vi "TA for 3.0.vi"(0 "Folder Name":string, 1 "Name of File":string, 2 "Folder to Save":path, 3 "Timepoints":dbl[](array[numeric]), 4 "Vx array":dbl, 5 "Vy array":dbl) -> ()   [LabVIEW 2015]
uses:
  <vilib>/Utility/file.llb/Read Delimited Spreadsheet (DBL).vi
  <vilib>/Utility/file.llb/Write Delimited Spreadsheet (DBL).vi
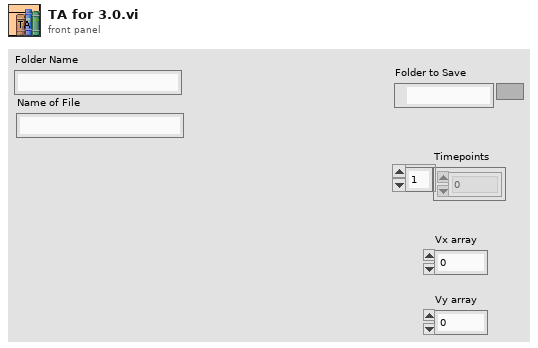
[diagram p1: front panel]
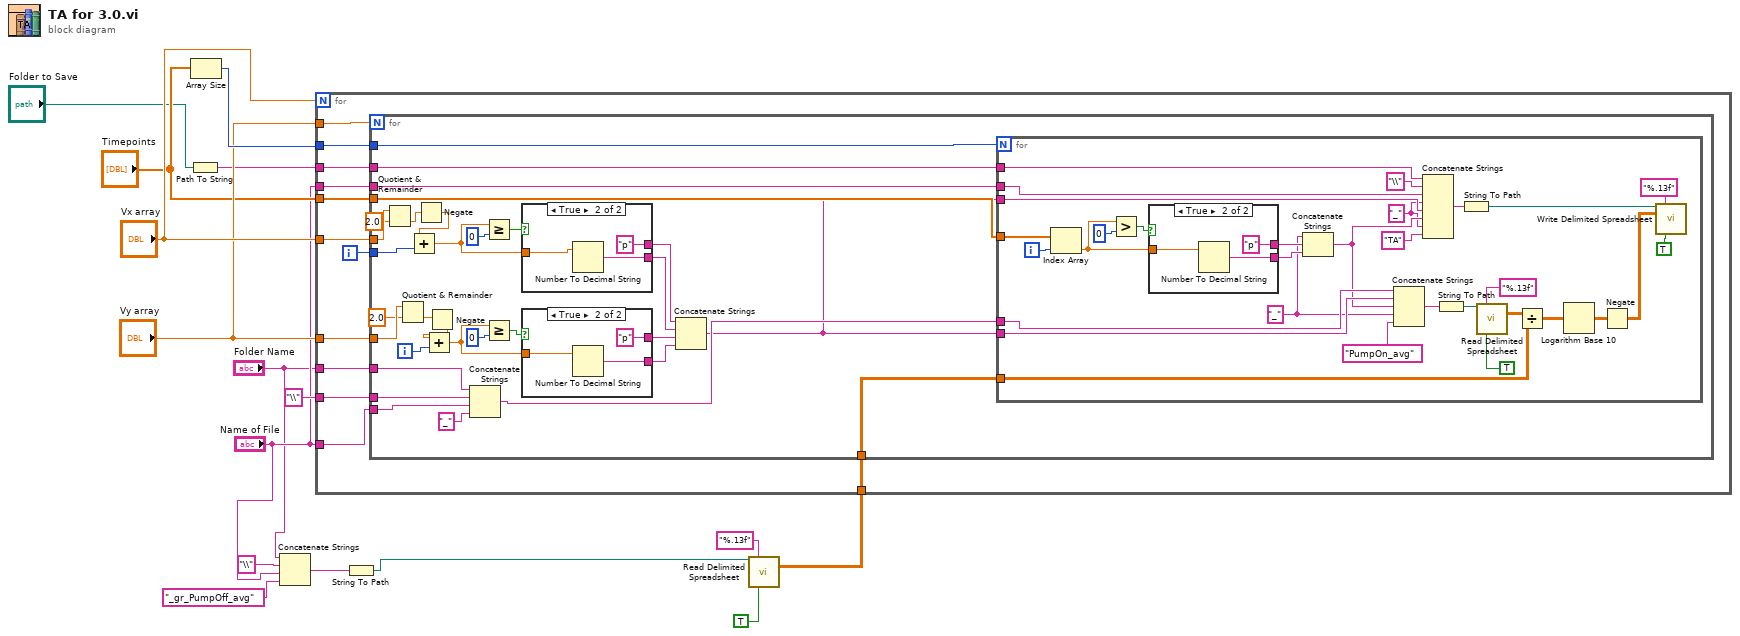
[diagram p0: block diagram]
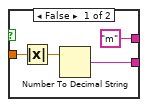
[diagram p2: hidden frame]
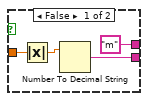
[diagram p3: hidden frame]
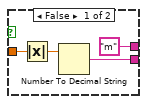
[diagram p4: hidden frame]
diagram:
  n1 = Path To String(path="Folder to Save") -> (string=w11:string)
  n2 = Array Size(array="Timepoints") -> (size(s)=w15:i32)
  n3 = Concatenate Strings("Folder Name", "\\" ("string"), "Name of File", "_gr_PumpOff_avg" ("string")) -> (w3:string)
  n4 = String To Path(string=w3) -> (path=w2:path)
  n5 = call-poly <vilib>:"Read Delimited Spreadsheet.vi"("file path (dialog if empty)"=w2, "format (%.3f)"="%.13f", "transpose? (F)"=TRUE) -> ("all rows"=w8:dbl[][])  [unwired: 7 in, 5 out]
  n6 = for {
    N: "Vx array" -> [_]
    tunnel: "Name of File" -> [w28]
    tunnel: "\\" -> [w27]
    tunnel: "Folder Name" -> [w26]
    tunnel: "Vy array" -> [w25]
    tunnel: w15 -> [w24]
    tunnel: "Vx array" -> [w23]
    tunnel: "Vy array" -> [w21]
    tunnel: "Timepoints" -> [w20]
    tunnel: w11 -> [w19]
    tunnel: "Name of File" -> [w18]
    tunnel: w8 -> [w17]
    i -> [w22]
    n7 = for {
      N: w25 -> [_]
      tunnel: w28 -> [w38]
      tunnel: w27 -> [w39]
      tunnel: w26 -> [w59]
      tunnel: w24 -> [w58]
      tunnel: w23 -> [w36]
      tunnel: w22 -> [w55]
      tunnel: w21 -> [w32]
      tunnel: w20 -> [w45]
      tunnel: w19 -> [w44]
      tunnel: w18 -> [w43]
      tunnel: w17 -> [w37]
      i -> [w50]
      n8 = Quotient & Remainder(x=w36, y=2.0) -> (floor(x/y)=w34:dbl)  [unwired: 1 out]
      n9 = Quotient & Remainder(x=w32, y=2.0) -> (floor(x/y)=w30:dbl)  [unwired: 1 out]
      n10 = Negate(x=w34) -> (-x=w33:dbl)
      n11 = Add(x=w33, y=w55) -> (x+y=w54:dbl)
      n12 = Negate(x=w30) -> (-x=w29:dbl)
      n13 = Add(x=w29, y=w50) -> (x+y=w51:dbl)
      n14 = Concatenate Strings(w59, w39, w38, "_") -> (w41:string)
      n15 = Greater Or Equal?(x=w54, y=0) -> (x >= y?=w56:bool)
      n16 = Greater Or Equal?(x=w51, y=0) -> (x >= y?=w53:bool)
      n17 = case shown="True" w56 {
        tunnel: ["m" "p"] -> w49
        tunnel: w54 -> [w69 w71]
        tunnel: [w67 w72] -> w48
        frame False {
          n18 = Absolute Value(x=w69) -> (abs(x)=w68:dbl)
          n19 = Number To Decimal String(number=w68) -> (decimal integer string=w67:string)  [unwired: 1 in]
        }
        frame True {
          n20 = Number To Decimal String(number=w71) -> (decimal integer string=w72:string)  [unwired: 1 in]
        }
      }
      n21 = case shown="True" w53 {
        tunnel: ["m" "p"] -> w47
        tunnel: w51 -> [w62 w64]
        tunnel: [w60 w65] -> w46
        frame False {
          n22 = Absolute Value(x=w62) -> (abs(x)=w61:dbl)
          n23 = Number To Decimal String(number=w61) -> (decimal integer string=w60:string)  [unwired: 1 in]
        }
        frame True {
          n24 = Number To Decimal String(number=w64) -> (decimal integer string=w65:string)  [unwired: 1 in]
        }
      }
      n25 = Concatenate Strings(w49, w48, w47, w46) -> (w40:string)
      n26 = for {
        N: w58 -> [_]
        tunnel: w45 -> [w101]
        tunnel: w44 -> [w96]
        tunnel: w43 -> [w93]
        tunnel: w41 -> [w87]
        tunnel: w40 -> [w86]
        tunnel: w37 -> [w77]
        tunnel: w40 -> [w83]
        i -> [w100]
        w85 = "_"
        w81 = "_" ("string")
        n27 = Index Array(array=w101, index=w100) -> (element=w103:dbl)
        n28 = Greater?(x=w103, y=0) -> (0:w102:bool)
        n29 = case shown="True" w102 {
          tunnel: ["m" "p"] -> w98
          tunnel: w103 -> [w107 w109]
          tunnel: [w105 w110] -> w99
          frame False {
            n30 = Absolute Value(x=w107) -> (abs(x)=w106:dbl)
            n31 = Number To Decimal String(number=w106) -> (decimal integer string=w105:string)  [unwired: 1 in]
          }
          frame True {
            n32 = Number To Decimal String(number=w109) -> (decimal integer string=w110:string)  [unwired: 1 in]
          }
        }
        n33 = Concatenate Strings(w85, w98, w99) -> (w82:string)
        n34 = Concatenate Strings(w87, w86, w82, w85, "PumpOn_avg") -> (w89:string)
        n35 = Concatenate Strings(w96, "\\" ("string"), w93, w81, w83, w82, w81, "TA" ("string")) -> (w79:string)
        n36 = String To Path(string=w89) -> (path=w90:path)
        n37 = String To Path(string=w79) -> (path=w95:path)
        n38 = call-poly <vilib>:"Read Delimited Spreadsheet.vi"("file path (dialog if empty)"=w90, "format (%.3f)"="%.13f", "transpose? (F)"=TRUE) -> ("all rows"=w78:dbl[][])  [unwired: 7 in, 5 out]
        n39 = Divide(x=w78, y=w77) -> (x/y=w76:dbl[][])
        n40 = Logarithm Base 10(1:w76) -> (0:w75:dbl[][])
        n41 = Negate(x=w75) -> (-x=w74:dbl[][])
        n42 = call-poly <vilib>:"Write Delimited Spreadsheet.vi"("file path (dialog if empty)"=w95, "format (%.3f)"="%.13f", "2D data"=w74, "transpose? (F)"=TRUE) -> ()  [unwired: 10 in, 2 out]
      }
    }
  }
